vi "Configure Measurement.vi"(8 "error in (no error)":errorcluster, 10 "Measurement Name":string, 11 "Test Framework in":refnum<class "Test Framework.lvclass">) -> (0 "error out":errorcluster, 3 "Test Framework out":refnum<class "Test Framework.lvclass">)   [LabVIEW 2020, in "Test Framework.lvclass"]
doc: "Finds the measurement by name and configures it.\nWrites back all measurements after configuration to the class data."
uses:
  Test Framework.lvclass
  Test Framework.lvclass/Test Framework.ctl
  Measurements/Measurement.lvclass
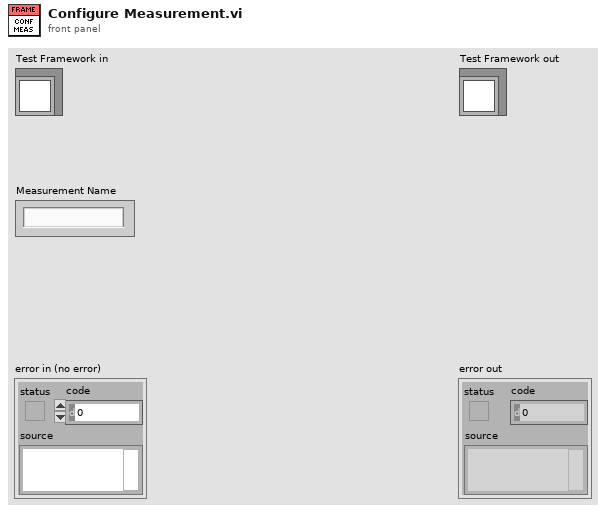
[diagram p1: front panel]
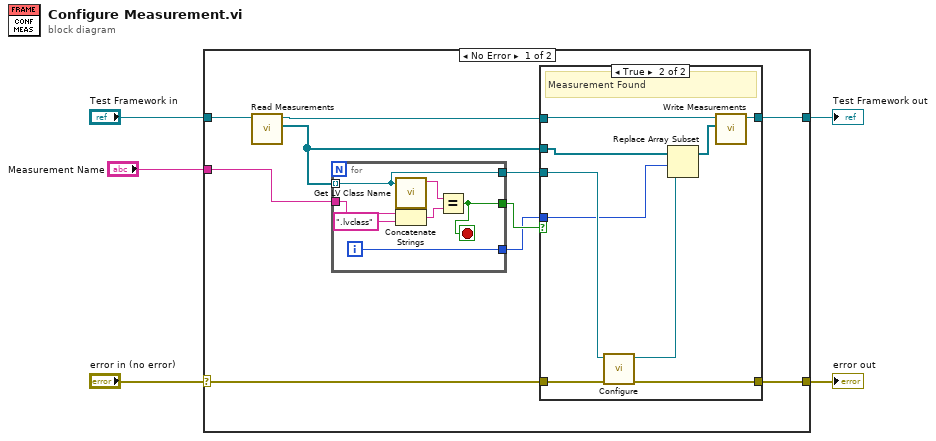
[diagram p0: block diagram]
diagram:
  n1 = case shown="No Error" "error in (no error)" {
    selector: "error in (no error)" -> [w11 w35]
    tunnel: [w10 w35] -> w4
    tunnel: [w7 w34] -> w2
    tunnel: "Test Framework in" -> [w15 w34]
    tunnel: "Measurement Name" -> [w14 _]
    frame No Error {
      n2 = call "Read Measurements.vi"("Test Framework in"=w15) -> ("Measurements"=w6:refnum<class "Measurement.lvclass">[], "Test Framework out"=w8:refnum<class "Test Framework.lvclass">)  [unwired: 9 in]
      n3 = for {
        tunnel: w6 -> [w29] mode=indexing
        tunnel: w14 -> [w33]
        tunnel: [w29] -> w12
        tunnel: [w28] -> w13
        tunnel: [w27] -> w9
        i -> [w27]
        stop <- w28 stop-if-true
        n4 = call <vilib>:"Get LV Class Name.vi"("object"=w29) -> ("class name"=w30:string)  [unwired: 9 in, 1 out]
        n5 = Concatenate Strings(w33, ".lvclass" ("string")) -> (w31:string)
        n6 = Equal?(x=w30, y=w31) -> (x = y?=w28:bool)
      }
      n7 = case shown="True" w13 {
        tunnel: w12 -> [_ w25]
        tunnel: w11 -> [w16 w26]
        tunnel: [w16 w24] -> w10
        tunnel: w9 -> [_ w22]
        tunnel: w8 -> [w17 w20]
        tunnel: [w17 w19] -> w7
        tunnel: w6 -> [_ w23]
        frame False {
        }
        frame True {
          # "Measurement Found"
          n8 = call-dynamic "Configure.vi"("error in (no error)"=w26, "Measurements in"=w25) -> ("error out"=w24:errorcluster, "Measurements out"=w21:refnum<class "Measurement.lvclass">)  [unwired: 8 in]
          n9 = Replace Array Subset(array=w23, new element=w21, index=w22) -> (w18:refnum<class "Measurement.lvclass">[])
          n10 = call "Write Measurements.vi"("Measurements"=w18, "Test Framework in"=w20) -> ("Test Framework out"=w19:refnum<class "Test Framework.lvclass">)  [unwired: 9 in]
        }
      }
    }
    frame Error {
    }
  }
  "error out" <- w4
  "Test Framework out" <- w2
